vi "Create Dynamic Member VI In LVClass.vi"(7 "RPC Method Name":string, 8 "error in (no error)":errorcluster, 9 "New VI Path":path=path "C:/Users/sujain/Desktop/test/abcMember.vi", 10 "Member VI Template Path":path=path "C:/Users/sujain/Desktop/test/MemberTemplate.vi", 11 "LVClassLibrary in":refnum<vi>) -> (0 "error out":errorcluster, 3 "dynamic member vi out":refnum<vi>)   [LabVIEW 2019, in "gRPC Template Creation Utility.lvlib"]
uses:
  gRPC Template Creation Utility.lvlib
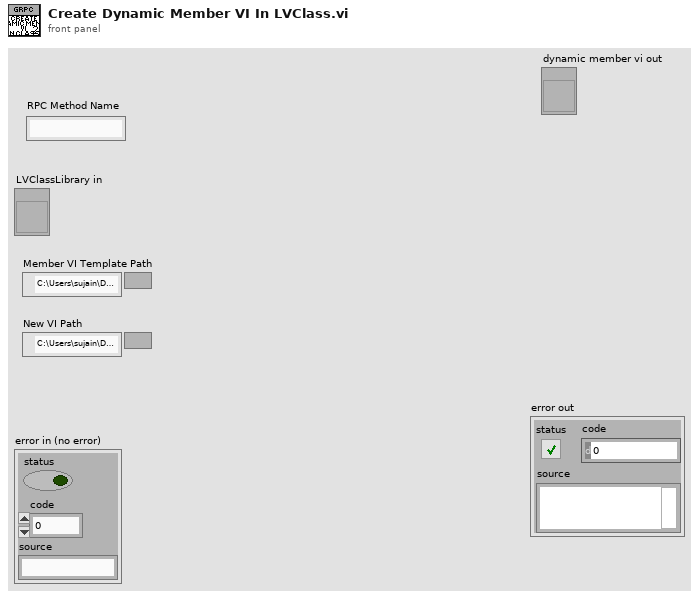
[diagram p1: front panel]
types:
  T1 = enum16{"Invalid Wire Rule", "Required", "Recommended", "Optional", "Dynamic Dispatch"}
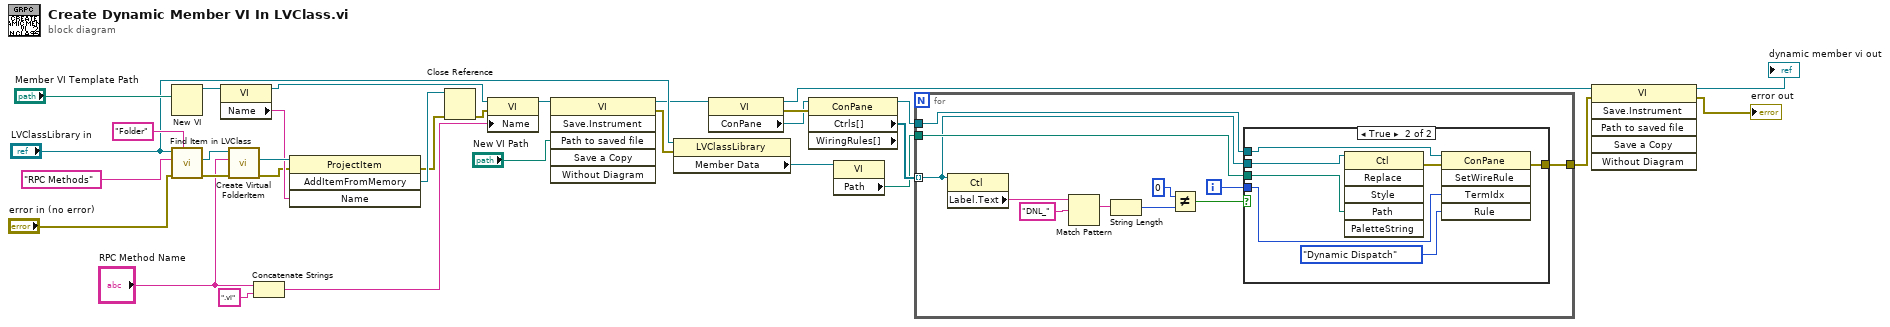
[diagram p0: block diagram]
diagram:
  n1 = New VI(10:"Member VI Template Path") -> (3:w18:refnum<vi>)  [unwired: 6 in, 1 out]
  n2 = call "Find Item in LVClass.vi"("Item Type"="Folder", "error in (no error)"="error in (no error)", "Item Name"="RPC Methods", "Class Item in"="LVClassLibrary in") -> ("error out"=w13:errorcluster, "Project Item (Class Item)"=w20:refnum<vi>)  [unwired: 4 in, 2 out]
  n3 = property class="VI"(reference=w18) -> (reference out=w7:refnum<vi>, "Name"=w17:string)  [unwired: 1 in, 1 out]
  n4 = call "Create Virtual FolderItem.vi"("error in (no error)"=w13, "Folder Name"="RPC Method Name", "ProjectItem in"=w20) -> ("error out"=w12:errorcluster, "FolderItem reference out"=w19:refnum<vi>)  [unwired: 5 in, 2 out]
  n5 = Concatenate Strings("RPC Method Name", ".vi" ("string")) -> (w8:string)
  n6 = invoke class="ProjectItem" method="AddItemFromMemory"(reference=w19, error in=w12, "Name"=w17) -> (error out=w15:errorcluster, "AddItemFromMemory"=w16:refnum<vi>)  [unwired: 1 in, 2 out]
  n7 = Close Reference(reference=w16, error in (no error)=w15) -> (error out=w11:errorcluster)
  n8 = property class="VI"(reference=w7, error in=w11, "Name"=w8) -> (reference out=w6:refnum<vi>)  [unwired: 1 out]
  n9 = invoke class="VI" method="Save.Instrument"(reference=w6, "Path to saved file"="New VI Path") -> (reference out=w3:refnum<vi>, error out=w4:errorcluster)  [unwired: 4 in, 4 out]
  n10 = property class="LVClassLibrary"(reference="LVClassLibrary in", error in=w4) -> ("Member Data"=w31:refnum<vi>)  [unwired: 2 out]
  n11 = property class="VI"(reference=w3) -> (reference out=w24:refnum<vi>, error out=w32:errorcluster, "ConPane"=w29:refnum<vi>)  [unwired: 1 in]
  n12 = property class="ConPane" props=["Ctrls[]", "WiringRules[]"](reference=w29, error in=w32) -> (reference out=w25:refnum<vi>, "Ctrls[]"=w27:refnum<vi>[])  [unwired: 2 out]
  n13 = property class="VI"(reference=w31) -> ("Path"=w26:path)  [unwired: 1 in, 2 out]
  n14 = for {
    tunnel: w27 -> [w39] mode=indexing
    tunnel: w26 -> [w43]
    tunnel: w25 -> [w42]
    tunnel: [w40] -> w23
    i -> [w41]
    n15 = property class="Ctl"(reference=w39) -> ("Label.Text"=w38:string)  [unwired: 1 in, 2 out]
    n16 = Match Pattern(string=w38, regular expression="DNL_") -> (match substring=w36:string)  [unwired: 1 in, 3 out]
    n17 = String Length(string=w36) -> (length=w35:i32)
    n18 = Not Equal?(x=0, y=w35) -> (x != y?=w33:bool)
    n19 = case shown="True" w33 {
      tunnel: w39 -> [_ w50]
      tunnel: w43 -> [_ w49]
      tunnel: w42 -> [_ w48]
      tunnel: w41 -> [_ w46]
      tunnel: [_ w44] -> w40
      frame False {
      }
      frame True {
        n20 = invoke class="Ctl" method="Replace"(reference=w50, "Path"=w49) -> (error out=w45:errorcluster)  [unwired: 4 in, 5 out]
        n21 = invoke class="ConPane" method="SetWireRule"(reference=w48, error in=w45, "TermIdx"=w46, "Rule"=T1."Dynamic Dispatch") -> (error out=w44:errorcluster)  [unwired: 1 in, 4 out]
      }
    }
  }
  n22 = invoke class="VI" method="Save.Instrument"(reference=w24, error in=w23) -> (reference out=→"dynamic member vi out":refnum<vi>, error out=→"error out":errorcluster)  [unwired: 4 in, 4 out]
